vi "Send experiment info.vi"(8 "error in (no error)":errorcluster, 11 "Tomo in":refnum<class "Tomo.lvclass">) -> (0 "error out":errorcluster, 3 "Tomo out":refnum<class "Tomo.lvclass">)   [LabVIEW 2012, in "Tomo.lvclass"]
uses:
  Tomo.lvclass
  <vilib>/Distrio/Murmex/Murmex/update_cluster.ctl
  volume map.ctl
  Tomo.lvclass/Tomo.ctl
  <vilib>/Distrio/Murmex/Murmex/Murmex.lvclass
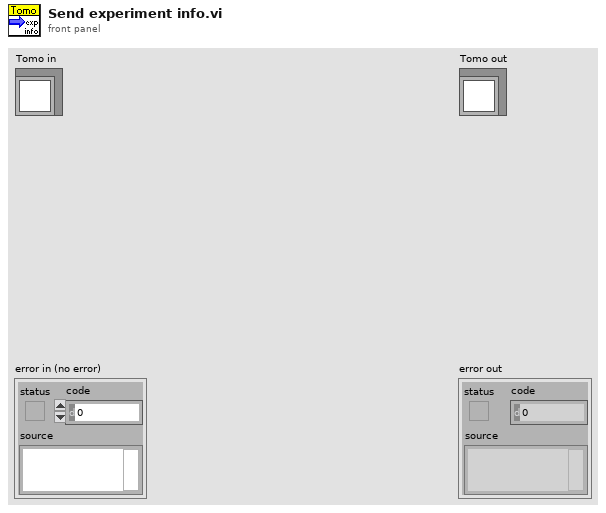
[diagram p1: front panel]
types:
  T1 = typedef "Tomo.lvclass/volume map.ctl" = enum16{"Cubic volume", "Custom volume", "Self-generate volume", "Time- tomography"}
  T2 = typedef "Murmex.lvlib/Murmex.lvclass/update_cluster.ctl" = cluster{"target ID":string, "key chains":string[], "values":variant[]}
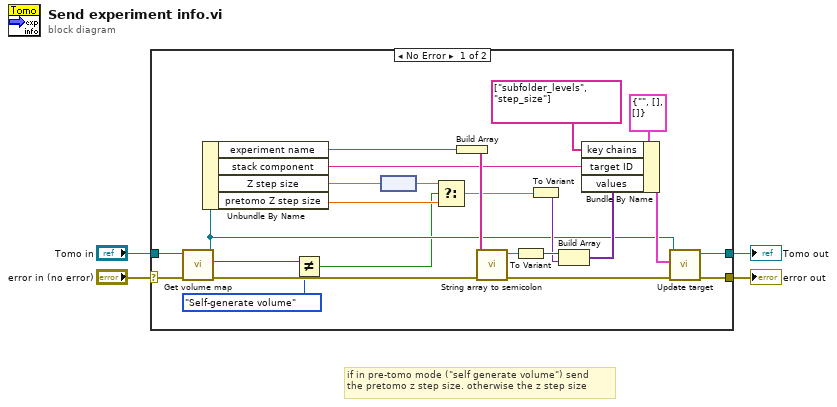
[diagram p0: block diagram]
diagram:
  # "if in pre-tomo mode (\"self generate volume\") send\nthe pretomo z step size. otherwise the z step size"
  n1 = case shown="No Error" "error in (no error)" {
    selector: "error in (no error)" -> [w14 w30]
    tunnel: [w15 w30] -> w3
    tunnel: [w16 w29] -> w1
    tunnel: "Tomo in" -> [w12 w29]
    frame No Error {
      n2 = call-dynamic "Get volume map.vi"("error in (no error)"=w14, "Tomo in"=w12) -> ("error out"=w13:errorcluster, "Volume map"=w10:T1, "Tomo out"=w11:refnum<class "Tomo.lvclass">)  [unwired: 7 in]
      n3 = Unbundle By Name(w11) -> ("experiment name"=w17:string, "stack component"=w25:string, "Z step size"=w20:dbl[unit], "pretomo Z step size"=w8:dbl[unit])
      n4 = Not Equal?(x=w10, y=volume_map."Self-generate volume") -> (x != y?=w7:bool)
      n5 = node(w20) -> (w6:dbl)
      n6 = Select(t=w6, s=w7, f=w8) -> (s? t:f=w5:dbl[unit])
      n7 = Build Array(w17) -> (w28:string[])
      n8 = call "String array to semicolon.vi"("error in"=w13, "String array"=w28) -> ("error out"=w26:errorcluster, "Semicolon string"=w19:string)  [unwired: 8 in]
      n9 = To Variant(anything=w19) -> (Variant=w24:variant)
      n10 = To Variant(anything=w5) -> (Variant=w18:variant)
      n11 = Build Array(w24, w18) -> (w23:variant[])
      n12 = Bundle By Name(cluster=T2 {"target ID"="", "key chains"=[], "values"=[]} ("update cluster"), "key chains"=string[] ["subfolder_levels", "step_size"], "target ID"=w25, "values"=w23) -> (w22:T2)
      n13 = call <vilib>:"Update target.vi"("error in (no error)"=w26, "update cluster"=w22, "MurmexBase in"=w11) -> ("error out"=w15:errorcluster, "MurmexBase out"=w16:refnum<class "Tomo.lvclass">)  [unwired: 7 in]
    }
    frame Error {
    }
  }
  "error out" <- w3
  "Tomo out" <- w1
